vi "Turn Off All Outputs.vi"(8 "error in (no error)":errorcluster, 11 "NI-DAQ in":refnum<class "NI-DAQ.lvclass">) -> (0 "error out":errorcluster, 3 "NI-DAQ out":refnum<class "NI-DAQ.lvclass">)   [LabVIEW 2016, in "NI-DAQ.lvclass"]
uses:
  NI-DAQ.lvclass
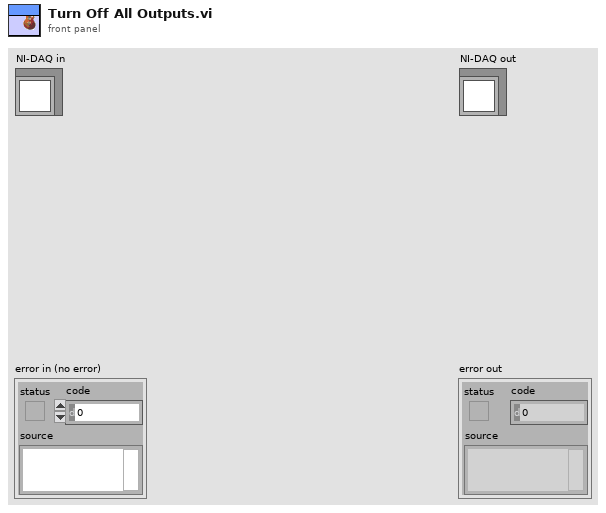
[diagram p1: front panel]
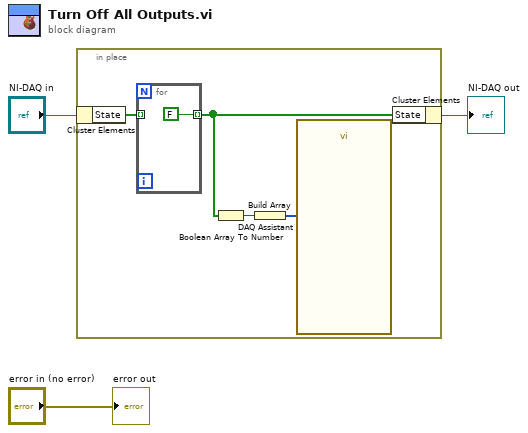
[diagram p0: block diagram]
diagram:
  n1 = in-place {
    n2 = in-place-cluster #1("NI-DAQ in") -> ("State"=w7:bool[])
    n3 = for {
      tunnel: w7 -> [_] mode=indexing
      tunnel: [FALSE] -> w4 mode=indexing
    }
    n4 = Boolean Array To Number(Boolean array=w4) -> (number=w6:u32)
    n5 = Build Array(w6) -> (w5:u32[])
    n6 = call "DAQ Assistant"("data"=w5) -> ()  [unwired: 17 in, 2 out]
    n7 = in-place-cluster #1("State"=w4) -> (→"NI-DAQ out":refnum<class "NI-DAQ.lvclass">)
  }
  "error out" <- "error in (no error)"
